vi "PID-Speed-Cntls.vi"(9 "ESTOP":bool, 10 "PID IN":dbl, 11 "Target Speed (m/s)":dbl) -> (3 "output":dbl)   [LabVIEW 2025]
uses:
  <vilib>/addons/control/pid/pid.llb/PID (DBL).vi
  <vilib>/addons/control/pid/NI_PID_pid.lvlib
panel:
  # "See block diagram for more information"
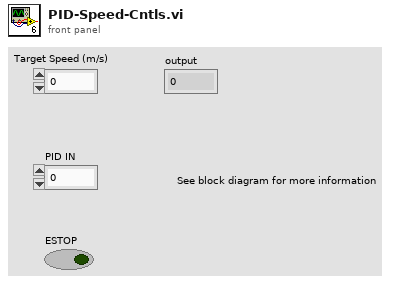
[diagram p1: front panel]
types:
  T1 = cluster{"proportional gain (Kc)":dbl, "integral time (Ti, min)":dbl, "derivative time (Td, min)":dbl}
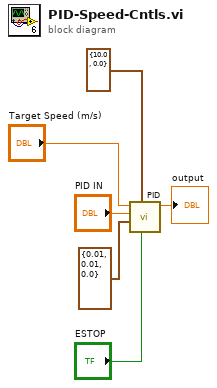
[diagram p0: block diagram]
diagram:
  n1 = call-poly <vilib>:"PID.vi"("reinitialize? (F)"="ESTOP", "output range"=cluster{"output high":dbl, "output low":dbl} {"output high"=10.0, "output low"=0.0}, "PID gains"=T1 {"proportional gain (Kc)"=0.01, "integral time (Ti, min)"=0.01, "derivative time (Td, min)"=0.0}, "process variable"="PID IN", "setpoint"="Target Speed (m/s)") -> ("output"=→"output":dbl)  [unwired: 5 in, 1 out]
